vi "Get Write Timeout.vi"(11 "Reply Protocol Base in":refnum<class "Reply Protocol Base.lvclass">) -> (2 "Write Timeout":i32=-1 format="%.0f ms", 3 "Reply Protocol Base out":refnum<class "Reply Protocol Base.lvclass">)   [LabVIEW 2023, in "HAL GOOP4.lvlib" / "Reply Protocol Base.lvclass"]
uses:
  Reply Protocol Base.lvclass
  Reply Protocol Base.lvclass/Reply Protocol Base.ctl
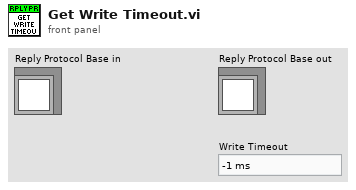
[diagram p1: front panel]
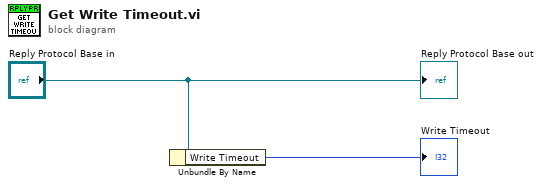
[diagram p0: block diagram]
diagram:
  n1 = Unbundle By Name("Reply Protocol Base in") -> ("Write Timeout"=→"Write Timeout":i32)
  "Reply Protocol Base out" <- "Reply Protocol Base in"
